vi "Fit Transform.vi"(7 "Type X":T1(ring), 8 "error in (no error)":errorcluster caption="entrée d'erreur (pas d'erreur)", 9 "y":string[][](array[string]), 10 "X":string[][](array[string]), 11 "QuantileTransformer.lvclass":refnum<class "QuantileTransformer.lvclass">) -> (0 "error out":errorcluster caption="sortie d'erreur", 2 "Data":T2, 3 "QuantileTransformer.lvclass":refnum<class "QuantileTransformer.lvclass">)   [LabVIEW 2020, in "QuantileTransformer.lvclass"]
doc: "Fit to data, then transform it.\n\nFits transformer to X and y with optional parameters fit_params and returns a transformed version of X.\n\nReturns : \n\n- X_new : ndarray array of shape (n_samples, n_features_new)\nTransformed array."
uses:
  QuantileTransformer.lvclass
  QuantileTransformer.lvclass/QuantileTransformer.ctl
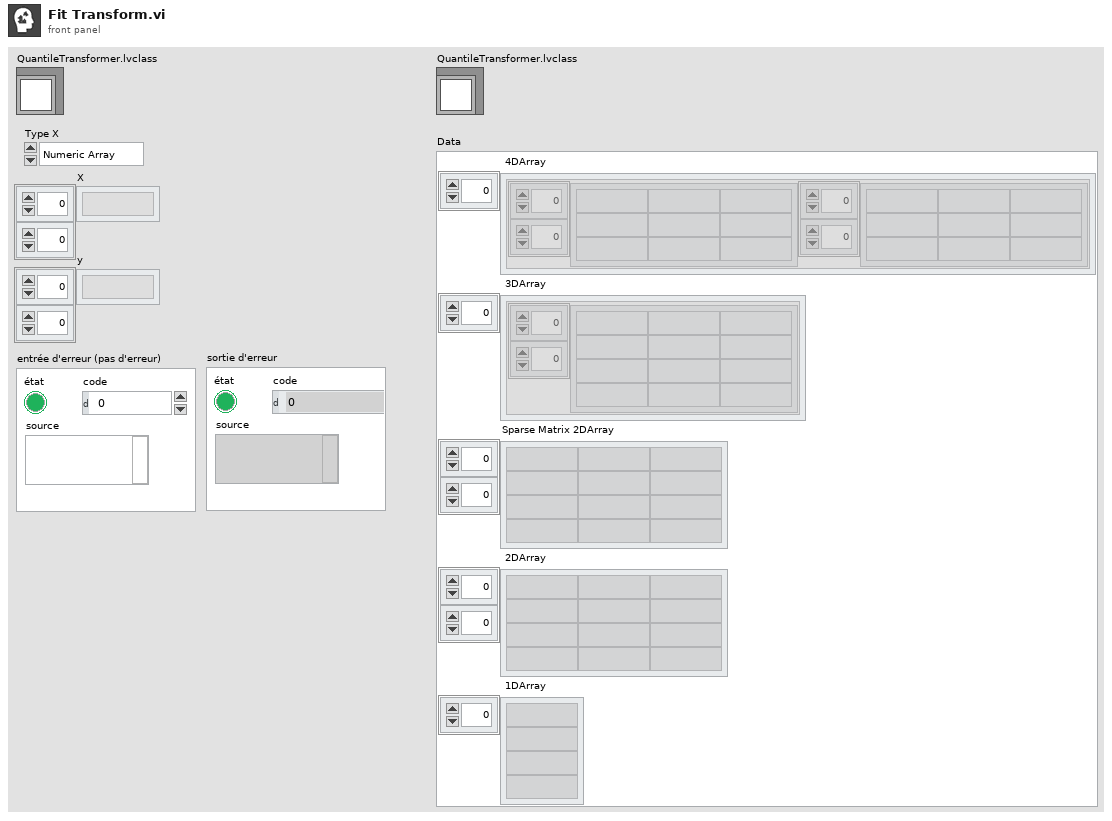
[diagram p1: front panel]
types:
  T1 = enum16{"Numeric Array", "String Array", "Sparse"}
  T2 = cluster{" 4DArray":cluster{"1":string[][], "2":string[][]}[], " 3DArray":cluster{"Tableau":string[][]}[], "Sparse Matrix 2DArray":string[][], " 2DArray":string[][], " 1DArray":string[]}
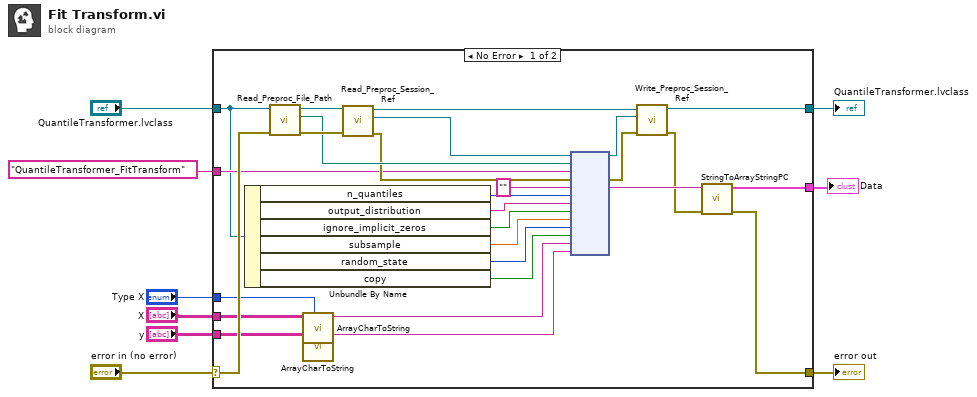
[diagram p0: block diagram]
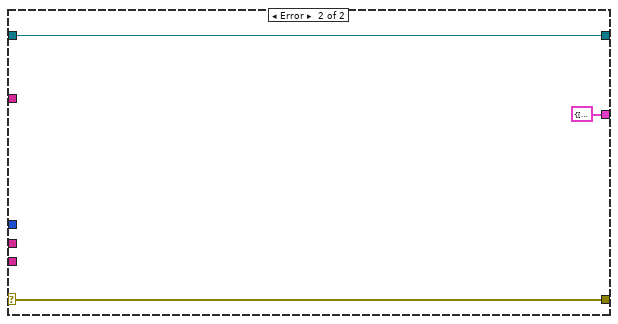
[diagram p2: hidden frame]
diagram:
  n1 = case shown="No Error" "error in (no error)" {
    selector: "error in (no error)" -> [w25 w40]
    tunnel: [w10 w40] -> w8
    tunnel: [w12 w39] -> w6
    tunnel: "QuantileTransformer.lvclass" -> [w23 w39]
    tunnel: "QuantileTransformer_FitTransform" ("Fonction") -> [w24 _]
    tunnel: [w11 T2 {" 4DArray"=[], " 3DArray"=[], "Sparse Matrix 2DArray"=[], " 2DArray"=[], " 1DArray"=[]} ("Data")] -> w1
    tunnel: "X" -> [w19 _]
    tunnel: "y" -> [w18 _]
    tunnel: "Type X" -> [w17 _]
    frame No Error {
      n2 = Unbundle By Name(w23) -> ("n_quantiles"=w28:i32, "output_distribution"=w27:string, "ignore_implicit_zeros"=w26:bool, "subsample"=w22:dbl, "random_state"=w21:i32, "copy"=w20:bool)
      n3 = call-dynamic "Read_Preproc_File_Path.vi"("error in (no error)"=w25, "Python in"=w23) -> ("error out"=w36:errorcluster, "File_Path"=w33:path, "Python out"=w37:refnum<class "QuantileTransformer.lvclass">)  [unwired: 7 in]
      n4 = call "ArrayCharToString.vi"("Type"=w17, "TAB"=w19) -> ("Instruction"=w16:string)  [unwired: 9 in]
      n5 = call "ArrayCharToString.vi"("TAB"=w18) -> ("Instruction"=w15:string)  [unwired: 10 in]
      n6 = call-dynamic "Read_Preproc_Session_Ref.vi"("error in (no error)"=w36, "Python in"=w37) -> ("error out"=w32:errorcluster, "Session_ref"=w34:refnum<k35>, "Python out"=w35:refnum<class "QuantileTransformer.lvclass">)  [unwired: 7 in]
      n7 = node(w34, w33, w24, w32, "", w28, w27, w26, w22, w21, w20, w16, w15) -> (w30:refnum<k35>, w31:errorcluster, w14:string)  [unwired: 8 in, 2 out]
      n8 = call-dynamic "Write_Preproc_Session_Ref.vi"("error in (no error)"=w31, "Session_ref"=w30, "Python in"=w35) -> ("error out"=w13:errorcluster, "Python out"=w12:refnum<class "QuantileTransformer.lvclass">)  [unwired: 7 in]
      n9 = call "StringToArrayStringPC.vi"("sortie d'erreur"=w13, "Return value"=w14) -> ("sortie d'erreur"=w10:errorcluster, "Data"=w11:T2)  [unwired: 8 in]
    }
    frame Error {
    }
  }
  "error out" <- w8
  "QuantileTransformer.lvclass" <- w6
  "Data" <- w1
